vi "FRCts20_WebMethods_Request_DELETE.vi"(7 "httpRequestID":u32, 11 "request":string) -> ()   [LabVIEW 2013, in "FRCts20_WebMethods.lvlib"]
doc: "<B>DELETE</B> the specified <B>request</B> resource\n\nhttp://<server address>:<port>/FRCts/request/<B>request</B>\n\n{requires authentication}"
uses:
  FRCts20_WebMethods.lvlib
  Backend/source/VI Source/FRCts20_Backend_API/FRCts20_Backend_API_Request.ctl
  Backend/source/VI Source/FRCts20_Backend_API/FRCts20_Backend_API_Status.ctl
  Backend/source/VI Source/FRCts20_Backend_API/FRCts20_Backend_API_Command_Request.ctl
  Backend/source/VI Source/FRCts20_Backend_API/FRCts20_Backend_API_Request.vi
  Backend/source/VI Source/FRCts20_Backend_API/FRCts20_Backend_API.lvlib
  <vilib>/wsapi/NI_WebServices.lvlib
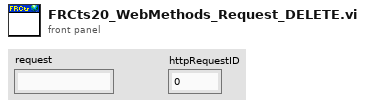
[diagram p1: front panel]
types:
  T1 = typedef "FRCts20_Backend_API.lvlib/FRCts20_Backend_API_Command_Request.ctl" = string
  T2 = typedef "FRCts20_Backend_API.lvlib/FRCts20_Backend_API_Request.ctl" = cluster{"Request Index":u32, "Description":string, "Status":T3, "Open Date":timestamp, "Last Update":timestamp, "Closed Date":timestamp, "Notes":cluster{"Note Index":u32, "Text":string, "Time Entered":timestamp, "Author":string, "Solution":bool}[], "Team Index":u32, "APIReturn":string}
  T3 = typedef "FRCts20_Backend_API.lvlib/FRCts20_Backend_API_Status.ctl" = enum16{"Open", "In Work", "Closed"}
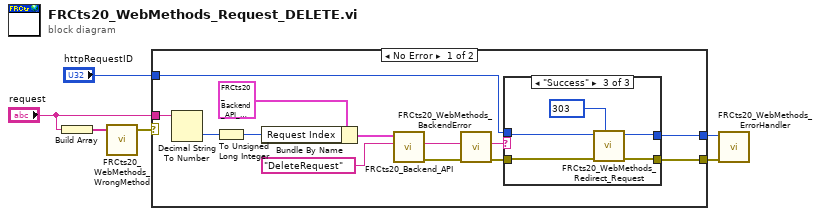
[diagram p0: block diagram]
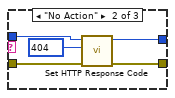
[diagram p3: hidden frame]
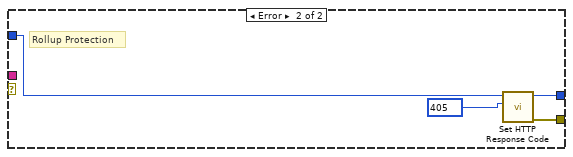
[diagram p4: hidden frame]
diagram:
  n1 = Build Array("request") -> (w2:string[])
  n2 = call "FRCts20_WebMethods_WrongMethod.vi"("Method Inputs"=w2) -> ("error out"=w1:errorcluster)  [unwired: 4 in]
  n3 = case shown="No Error" w1 {
    tunnel: "request" -> [w19 _]
    tunnel: [w15 w34] -> w6
    tunnel: "httpRequestID" -> [w14 w33]
    tunnel: [w16 w32] -> w3
    frame No Error {
      n4 = Decimal String To Number(string=w19) -> (number=w8:i32)  [unwired: 2 in, 1 out]
      n5 = To Unsigned Long Integer(number=w8) -> (unsigned 32bit integer=w7:u32)
      n6 = Bundle By Name(cluster=T2 {"Request Index"=0, "Description"="", "Status"=enum."Open", "Open Date"=timestamp(0 s since 1904-01-01), "Last Update"=timestamp(0 s since 1904-01-01), "Closed Date"=timestamp(0 s since 1904-01-01), "Notes"=[], "Team Index"=0, "APIReturn"=""} ("Request In"), "Request Index"=w7) -> (w17:T2)
      n7 = call-poly "FRCts20_Backend_API.vi"("Command"=T1 "DeleteRequest", "Request In"=w17) -> ("error out"=w13:errorcluster, "Status"=w12:string)  [unwired: 7 in, 1 out]
      n8 = call "FRCts20_WebMethods_BackendError.vi"("error in (no error)"=w13, "Status"=w12) -> ("error out"=w11:errorcluster, "Status out"=w10:string)  [unwired: 8 in]
      n9 = case shown="\"Success\"" w10 {
        tunnel: [w20 w25 w28] -> w16
        tunnel: [w21 w26 w31] -> w15
        tunnel: w14 -> [w20 w23 w29]
        tunnel: w11 -> [w21 w24 w30]
        frame "Backend Error", Default {
        }
        frame "No Action" {
          w22 = 404 items=["100"=100, "101"=101, "200"=200, "201"=201, "202"=202, "203"=203, "204"=204, "205"=205, "206"=206, "300"=300, "301"=301, "302"=302, "303"=303, "304"=304, "305"=305, "306"=306, "307"=307, "400"=400, "401"=401, "402"=402, "403"=403, "404"=404, "405"=405, "406"=406, "407"=407, "408"=408, "409"=409, "410"=410, "411"=411, "412"=412, "413"=413, "414"=414, "415"=415, "416"=416, "417"=417, "500"=500, "501"=501, "502"=502, "503"=503, "504"=504, "505"=505] ("response code (200)")
          n10 = call <vilib>:"Set HTTP Response Code.vi"("error in (no error)"=w24, "response code (200)"=w22, "httpRequestID"=w23) -> ("error out"=w26:errorcluster, "httpRequestID out"=w25:u32)  [unwired: 7 in]
        }
        frame "Success" {
          w27 = 303 items=["100"=100, "101"=101, "200"=200, "201"=201, "202"=202, "203"=203, "204"=204, "205"=205, "206"=206, "300"=300, "301"=301, "302"=302, "303"=303, "304"=304, "305"=305, "306"=306, "307"=307, "400"=400, "401"=401, "402"=402, "403"=403, "404"=404, "405"=405, "406"=406, "407"=407, "408"=408, "409"=409, "410"=410, "411"=411, "412"=412, "413"=413, "414"=414, "415"=415, "416"=416, "417"=417, "500"=500, "501"=501, "502"=502, "503"=503, "504"=504, "505"=505] ("response code (200)")
          n11 = call "FRCts20_WebMethods_Redirect_Request.vi"("response code (200)"=w27, "error in (no error)"=w30, "httpRequestID"=w29) -> ("error out"=w31:errorcluster, "httpRequestID out"=w28:u32)  [unwired: 7 in]
        }
      }
    }
    frame Error {
      w35 = 405 items=["100"=100, "101"=101, "200"=200, "201"=201, "202"=202, "203"=203, "204"=204, "205"=205, "206"=206, "300"=300, "301"=301, "302"=302, "303"=303, "304"=304, "305"=305, "306"=306, "307"=307, "400"=400, "401"=401, "402"=402, "403"=403, "404"=404, "405"=405, "406"=406, "407"=407, "408"=408, "409"=409, "410"=410, "411"=411, "412"=412, "413"=413, "414"=414, "415"=415, "416"=416, "417"=417, "500"=500, "501"=501, "502"=502, "503"=503, "504"=504, "505"=505] ("response code (200)")
      # "Rollup Protection"
      n12 = call <vilib>:"Set HTTP Response Code.vi"("response code (200)"=w35, "httpRequestID"=w33) -> ("error out"=w34:errorcluster, "httpRequestID out"=w32:u32)  [unwired: 8 in]
    }
  }
  n13 = call "FRCts20_WebMethods_ErrorHandler.vi"("error in"=w6, "httpRequestID"=w3) -> ()  [unwired: 9 in, 1 out]
